vi "Delta Linear movement.vi"(8 "error in (no error)":errorcluster, 9 "z0":dbl(slide) scale=-135.0..50.0, 10 "y0":dbl(slide) scale=-115.0..115.0, 11 "x0":dbl(slide) scale=-115.0..115.0) -> (0 "error out":errorcluster)   [LabVIEW 2019]
uses:
  math/Global 1.vi
panel:
  out "thetaZ":dbl
  out "thetaX":dbl
  out "thetaY":dbl
  out "non-existing point":bool
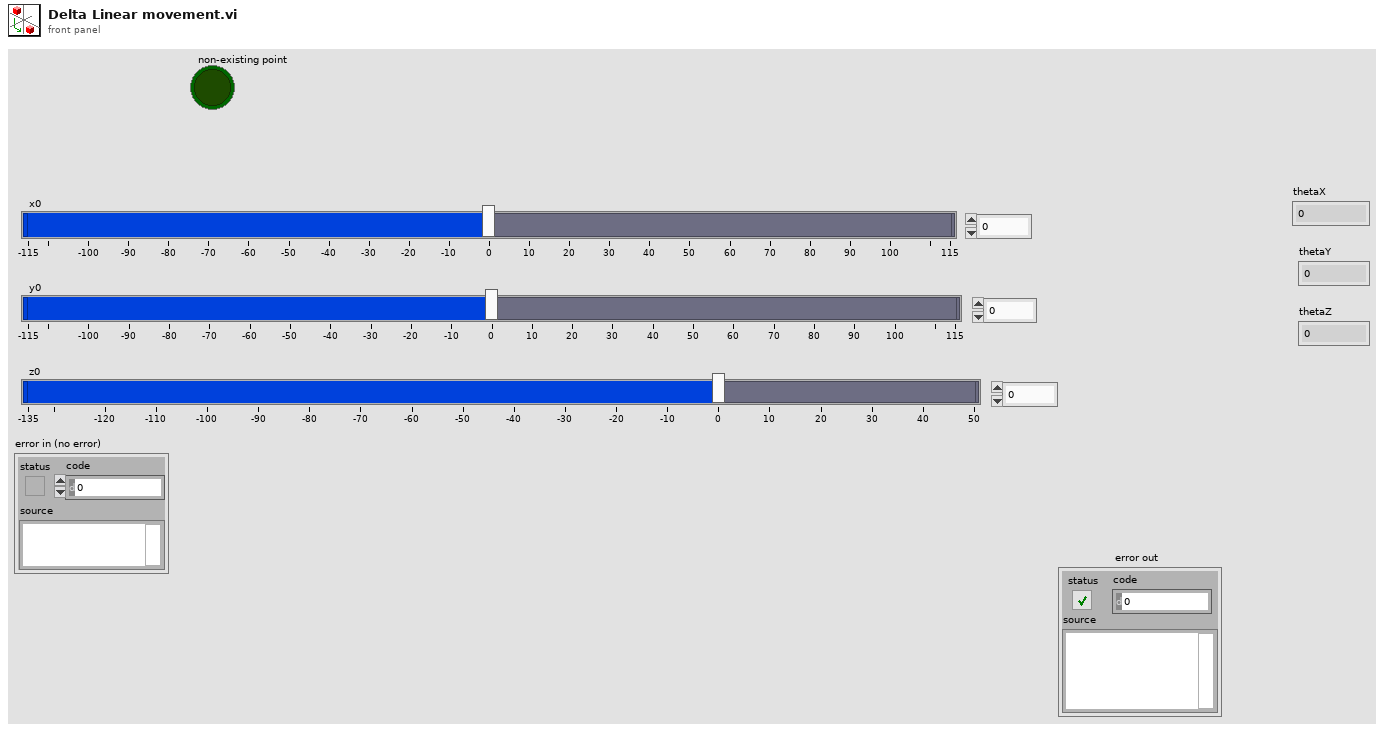
[diagram p1: front panel]
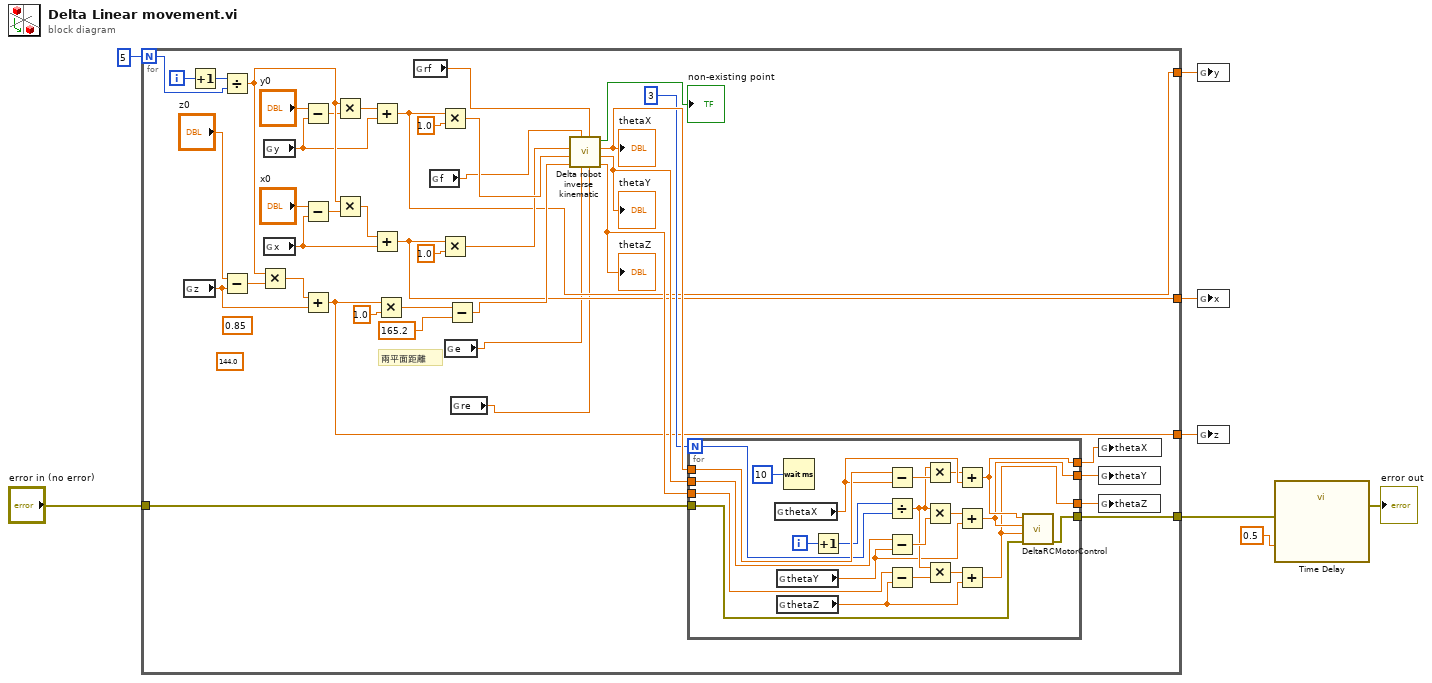
[diagram p0: block diagram]
diagram:
  n1 = for {
    N: 5 -> [w18]
    tunnel: [w34] -> w4
    tunnel: [w17] -> w7
    tunnel: [w16] -> w6
    tunnel: [w15] -> w5
    tunnel: "error in (no error)" -> [w14]
    i -> [w19]
    (unwired) 0.85 ("y")
    (unwired) 144.0 ("y")
    # "兩平面距離"
    n2 = global read "Global 1.vi" "z"() -> (w24:dbl)
    n3 = Increment(x=w19) -> (x+1=w26:i32)
    n4 = Divide(x=w26, y=w18) -> (x/y=w32:dbl)
    n5 = Subtract(x="z0", y=w24) -> (x-y=w33:dbl)
    n6 = Multiply(x=w32, y=w33) -> (x*y=w30:dbl)
    n7 = global read "Global 1.vi" "y"() -> (w22:dbl)
    n8 = global read "Global 1.vi" "x"() -> (w21:dbl)
    n9 = Subtract(x="y0", y=w22) -> (x-y=w31:dbl)
    n10 = Subtract(x="x0", y=w21) -> (x-y=w27:dbl)
    n11 = Add(x=w30, y=w24) -> (x+y=w15:dbl)
    n12 = Multiply(x=w32, y=w31) -> (x*y=w29:dbl)
    n13 = Multiply(x=w32, y=w27) -> (x*y=w28:dbl)
    n14 = Add(x=w29, y=w22) -> (x+y=w16:dbl)
    n15 = Add(x=w28, y=w21) -> (x+y=w17:dbl)
    n16 = Multiply(x=w15, y=1.0) -> (x*y=w36:dbl)
    n17 = global read "Global 1.vi" "rf"() -> (w13:dbl)
    n18 = global read "Global 1.vi" "f"() -> (w12:dbl)
    n19 = Multiply(x=w16, y=1.0) -> (x*y=w41:dbl)
    n20 = Multiply(x=w17, y=1.0) -> (x*y=w39:dbl)
    n21 = global read "Global 1.vi" "e"() -> (w11:dbl)
    n22 = Subtract(x=w36, y=165.2) -> (x-y=w35:dbl)
    n23 = global read "Global 1.vi" "re"() -> (w10:dbl)
    n24 = call "Delta robot inverse kinematic.vi"("re"=w10, "rf"=w13, "e"=w11, "f"=w12, "z0"=w35, "y0"=w41, "x0"=w39) -> ("thetaZ"=w47:dbl, "thetaY"=w48:dbl, "thetaX"=w49:dbl, "non-existing point"=→"non-existing point":bool)  [unwired: 1 in]
    "thetaZ" <- w47
    "thetaX" <- w49
    "thetaY" <- w48
    n25 = for {
      N: 3 -> [w64]
      tunnel: w49 -> [w70]
      tunnel: w48 -> [w69]
      tunnel: w47 -> [w68]
      tunnel: [w54] -> w45
      tunnel: [w52] -> w44
      tunnel: [w53] -> w43
      tunnel: w14 -> [w51]
      tunnel: [w50] -> w34
      i -> [w66]
      n26 = global read "Global 1.vi" "thetaX"() -> (w67:dbl)
      n27 = global read "Global 1.vi" "thetaY"() -> (w56:dbl)
      n28 = global read "Global 1.vi" "thetaZ"() -> (w55:dbl)
      n29 = Wait (ms)(milliseconds to wait=u32 10) -> ()  [unwired: 1 out]
      n30 = Increment(x=w66) -> (x+1=w65:i32)
      n31 = Subtract(x=w70, y=w67) -> (x-y=w63:dbl)
      n32 = Divide(x=w65, y=w64) -> (x/y=w58:dbl)
      n33 = Subtract(x=w69, y=w56) -> (x-y=w59:dbl)
      n34 = Subtract(x=w68, y=w55) -> (x-y=w57:dbl)
      n35 = Multiply(x=w58, y=w63) -> (x*y=w62:dbl)
      n36 = Multiply(x=w58, y=w59) -> (x*y=w61:dbl)
      n37 = Multiply(x=w58, y=w57) -> (x*y=w60:dbl)
      n38 = Add(x=w62, y=w67) -> (x+y=w54:dbl)
      n39 = Add(x=w61, y=w56) -> (x+y=w53:dbl)
      n40 = Add(x=w60, y=w55) -> (x+y=w52:dbl)
      n41 = call "DeltaRCMotorControl.vi"("error in (no error)"=w51, "Theta3"=w52, "Theta2"=w53, "Theta1"=w54) -> ("error out"=w50:errorcluster)  [unwired: 7 in]
    }
    n42 = global write "Global 1.vi" "thetaX"(w45) -> ()
    n43 = global write "Global 1.vi" "thetaY"(w43) -> ()
    n44 = global write "Global 1.vi" "thetaZ"(w44) -> ()
  }
  n45 = global write "Global 1.vi" "y"(w6) -> ()
  n46 = global write "Global 1.vi" "x"(w7) -> ()
  n47 = global write "Global 1.vi" "z"(w5) -> ()
  n48 = call "Time Delay"("error in (no error)"=w4, "Delay Time (s)"=0.5) -> ("error out"=→"error out":errorcluster)  [unwired: 9 in]
